vi "Read Tab Location.vi"(9 "Tab in":refnum<class "Tab.lvclass">) -> (3 "Tab out":refnum<class "Tab.lvclass">, 4 "Tab Location":enum32{"Top", "Bottom", "Left", "Right"}(ring))   [LabVIEW 2014, in "Tab.lvclass"]
uses:
  Tab.lvclass
  Tab.lvclass/Tab.ctl
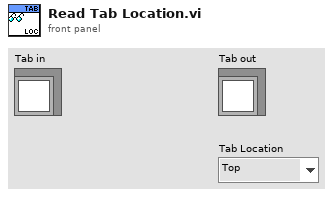
[diagram p1: front panel]
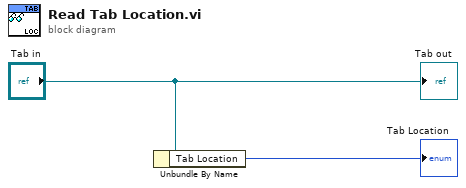
[diagram p0: block diagram]
diagram:
  n1 = Unbundle By Name("Tab in") -> ("Tab Location"=→"Tab Location":enum32{"Top", "Bottom", "Left", "Right"})
  "Tab out" <- "Tab in"
